vi "FormatData.vi"(11 "Raw data":u64[](array[numeric])) -> (3 "Scaled":dbl[][](array[numeric]))   [LabVIEW 2013, in "FpgaRef5782.lvclass"]
uses:
  FpgaRef5782.lvclass
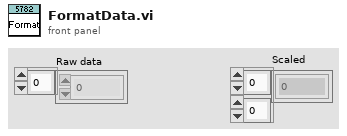
[diagram p1: front panel]
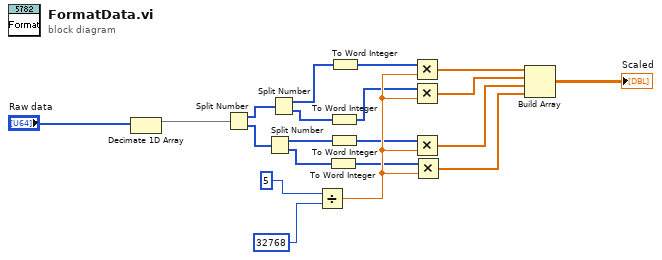
[diagram p0: block diagram]
diagram:
  n1 = Decimate 1D Array("Raw data") -> (w6:u64[])  [unwired: 1 out]
  n2 = Split Number(x=w6) -> (hi(x)=w11:u32[], lo(x)=w15:u32[])
  n3 = Split Number(x=w15) -> (hi(x)=w13:u16[], lo(x)=w12:u16[])
  n4 = Split Number(x=w11) -> (hi(x)=w10:u16[], lo(x)=w14:u16[])
  n5 = Divide(x=5, y=32768) -> (x/y=w20:dbl)
  n6 = To Word Integer(number=w12) -> (16bit integer=w19:i16[])
  n7 = To Word Integer(number=w14) -> (16bit integer=w17:i16[])
  n8 = To Word Integer(number=w13) -> (16bit integer=w18:i16[])
  n9 = To Word Integer(number=w10) -> (16bit integer=w16:i16[])
  n10 = Multiply(x=w16, y=w20) -> (x*y=w5:dbl[])
  n11 = Multiply(x=w17, y=w20) -> (x*y=w4:dbl[])
  n12 = Multiply(x=w18, y=w20) -> (x*y=w3:dbl[])
  n13 = Multiply(x=w19, y=w20) -> (x*y=w2:dbl[])
  n14 = Build Array(w5, w4, w3, w2) -> (→"Scaled":dbl[][])
